vi "viewConfigText.vi"(8 "error in (no error)":errorcluster, 10 "prevName":string caption="default name", 11 "ConfigXMLControls":T1) -> (0 "error out":errorcluster)   [LabVIEW 2015]
uses:
  ConfigXMLControl.ctl
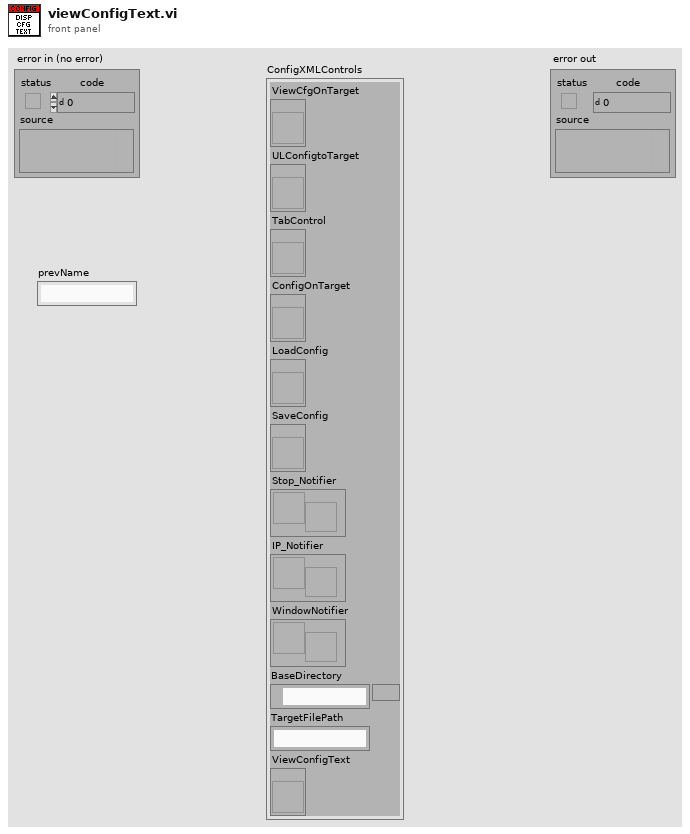
[diagram p1: front panel]
types:
  T1 = typedef "ConfigXMLControl.ctl" = cluster{"ViewCfgOnTarget":refnum<vi>, "ULConfigtoTarget":refnum<vi>, "TabControl":refnum<vi>, "ConfigOnTarget":refnum<vi>, "LoadConfig":refnum<vi>, "SaveConfig":refnum<vi>, "Stop_Notifier":refnum<notifier>, "IP_Notifier":refnum<notifier>, "WindowNotifier":refnum<notifier>, "BaseDirectory":path, "TargetFilePath":string, "ViewConfigText":refnum<vi>}
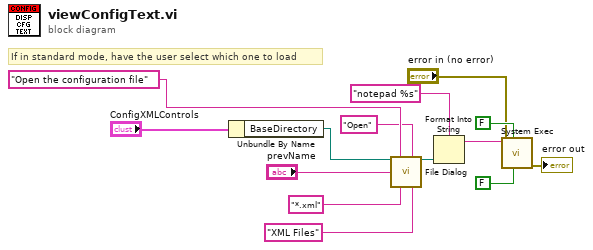
[diagram p0: block diagram]
diagram:
  # "If in standard mode, have the user select which one to load"
  n1 = Unbundle By Name("ConfigXMLControls") -> ("BaseDirectory"=w8:path)
  n2 = call "File Dialog"("start path"=w8, "prompt"="Open the configuration file", "button label"="Open", "default name"="prevName", "pattern (all files)"="*.xml", "pattern label"="XML Files") -> ("selected path"=w4:path)  [unwired: 6 in, 3 out]
  n3 = Format Into String(format string="notepad %s", w4) -> (resulting string=w3:string)  [unwired: 2 in, 1 out]
  n4 = call <vilib>:"System Exec.vi"("run minimized? (F)"=FALSE, "wait until completion? (T)"=FALSE, "error in (no error)"="error in (no error)", "command line"=w3) -> ("error out"=→"error out":errorcluster)  [unwired: 4 in, 3 out]
